vi "Add Initialization Block Diagram Content.vi"(8 "error in (no error)":errorcluster, 10 "Init":T1, 11 "EST Output in":refnum<class "EST Output.lvclass">) -> (0 "error out":errorcluster, 3 "EST Output out":refnum<class "EST Output.lvclass">)   [LabVIEW 2025, in "EST Output.lvclass"]
uses:
  EST Output.lvclass
  VI/VI/Init.Refs.ctl
  <vilib>/Utility/miscctls.llb/LVPointTypeDef.ctl
  <vilib>/_script/New VI Object TypeDefs/NewVIObject_LVRelativePositionTypeDef.ctl
  <vilib>/_script/New VI Object TypeDefs/NewVIObject_LVRelativeDirectionTypeDef.ctl
  <vilib>/Utility/miscctls.llb/LVPoint32TypeDef.ctl
  EST Output.lvclass/EST Output.ctl
  Signal/Read Signal Name.vi
  Read Memory Template Path.vi
  Read Load Path.vi
  VI/Structures/Structures.lvclass
  VI/VI/VI.lvclass
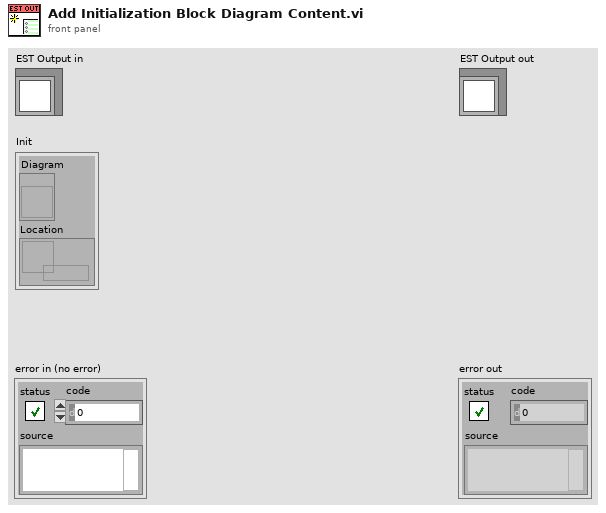
[diagram p1: front panel]
types:
  T1 = typedef "VI.lvclass/Init.Refs.ctl" = cluster{"Diagram":refnum<vi>, "Location":refnum<data-value>}
  T2 = typedef "NewVIObject_LVRelativePositionTypeDef.ctl" = cluster{"Refnum":refnum<vi>, "Relative Direction":T3, "Point32":T4}
  T3 = typedef "NewVIObject_LVRelativeDirectionTypeDef.ctl" = enum32{"Right", "Left", "Top", "Bottom", "Top Right", "Top Left", "Bottom Right", "Bottom Left"}
  T4 = typedef "LVPoint32TypeDef.ctl" = cluster{"Horizontal":i32, "Vertical":i32}
  T5 = typedef "LVPointTypeDef.ctl" = cluster{"Horizontal":i16, "Vertical":i16}
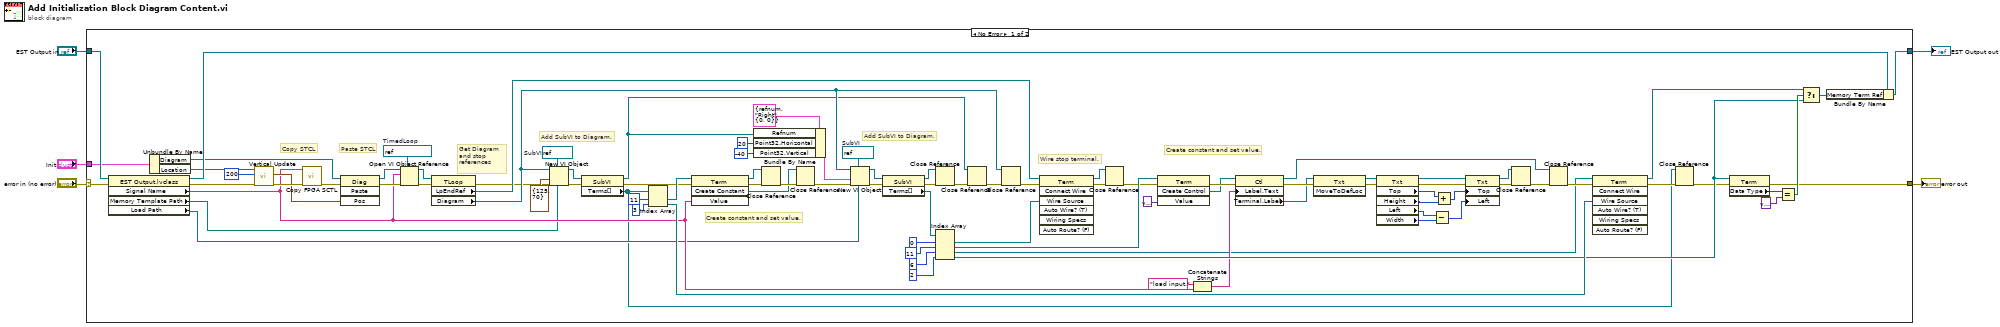
[diagram p0: block diagram]
diagram:
  n1 = case shown="No Error" "error in (no error)" {
    selector: "error in (no error)" -> [w59 w99]
    tunnel: "EST Output in" -> [w64 w100]
    tunnel: [w7 w99] -> w3
    tunnel: [w6 w100] -> w2
    tunnel: "Init" -> [w61 _]
    frame No Error {
      w55 = refnum<vi> refnum  # TimedLoop
      w89 = refnum<vi> refnum  # SubVI
      w84 = refnum<vi> refnum  # SubVI
      # "Create constant and set value."
      # "Wire stop terminal."
      # "Create constant and set value."
      # "Add SubVI to Diagram."
      # "Add SubVI to Diagram."
      # "Get Diagram and stop references"
      # "Paste STCL"
      # "Copy STCL"
      n2 = property class="EST Output.lvclass"(reference=w64, error in=w59) -> (reference out=w63:refnum<class "EST Output.lvclass">, error out=w45:errorcluster, "Signal Name"=w50:string, "Memory Template Path"=w42:path, "Load Path"=w43:path)
      n3 = Unbundle By Name(w61) -> ("Diagram"=w26:refnum<vi>, "Location"=w44:refnum<data-value>)
      n4 = call "Vertical Update.vi"("error in (no error)"=w45, "Vertical Change"=i16 200, "Location"=w44) -> ("error out"=w58:errorcluster, "location out"=w56:T5)  [unwired: 6 in, 1 out]
      n5 = call "Copy FPGA SCTL.vi"("error in (no error)"=w58, "SCTL Name"=w50) -> ("error out"=w57:errorcluster)  [unwired: 9 in]
      n6 = invoke class="Diag" method="Paste"(reference=w26, error in=w57, "Pos"=w56) -> (reference out=w54:refnum<vi>, error out=w53:errorcluster)  [unwired: 1 in, 2 out]
      n7 = Open VI Object Reference(7:w55, 8:w53, 10:w50, 11:w54) -> (0:w52:errorcluster, 3:w51:refnum<vi>)
      n8 = property class="TLoop"(reference=w51, error in=w52) -> (error out=w27:errorcluster, "LpEndRef"=w83:refnum<vi>, "Diagram"=w31:refnum<vi>)  [unwired: 1 out]
      n9 = New VI Object(vi object class=w84, owner refnum=w31, position/next to=T5 {"Horizontal"=125, "Vertical"=70} ("location"), 6:w42, 8:w27) -> (object refnum=w87:refnum<vi>, 0:w88:errorcluster)  [unwired: 3 in]
      n10 = property class="SubVI"(reference=w87, error in=w88) -> (reference out=w30:refnum<vi>, error out=w34:errorcluster, "Terms[]"=w36:refnum<vi>[])
      n11 = Index Array(array=w36, index #1=11 ("index"), index #2=3 ("index")) -> (element #1=w81:refnum<vi>, element #2=w82:refnum<vi>)
      n12 = invoke class="Term" method="Create Constant"(reference=w81, error in=w34, "Value"=w50) -> (reference out=w80:refnum<vi>, error out=w79:errorcluster, "Create Constant"=w76:refnum<vi>)  [unwired: 1 in, 1 out]
      n13 = Bundle By Name(cluster=T2 {"Refnum"=refnum, "Relative Direction"=enum."Right", "Point32"={"Horizontal"=0, "Vertical"=0}} ("Relative Position"), "Refnum"=w30, "Point32.Horizontal"=20, "Point32.Vertical"=-40) -> (w48:T2)
      n14 = Close Reference(reference=w80, error in (no error)=w79) -> (error out=w78:errorcluster)
      n15 = Close Reference(reference=w76, error in (no error)=w78) -> (error out=w77:errorcluster)
      n16 = New VI Object(vi object class=w89, owner refnum=w31, position/next to=w48, 6:w43, 8:w77) -> (object refnum=w91:refnum<vi>, 0:w90:errorcluster)  [unwired: 3 in]
      n17 = property class="SubVI"(reference=w91, error in=w90) -> (reference out=w75:refnum<vi>, error out=w74:errorcluster, "Terms[]"=w94:refnum<vi>[])
      n18 = Close Reference(reference=w75, error in (no error)=w74) -> (error out=w35:errorcluster)
      n19 = Index Array(array=w94, index #1=0 ("index"), index #2=11 ("index"), index #3=6 ("index"), index #4=2 ("index")) -> (element #1=w73:refnum<vi>, element #2=w72:refnum<vi>, element #3=w23:refnum<vi>, element #4=w67:refnum<vi>)
      n20 = Close Reference(reference=w30, error in (no error)=w35) -> (error out=w33:errorcluster)
      n21 = Close Reference(reference=w31, error in (no error)=w33) -> (error out=w32:errorcluster)
      n22 = invoke class="Term" method="Connect Wire"(reference=w83, error in=w32, "Wire Source"=w73) -> (reference out=w41:refnum<vi>, error out=w40:errorcluster)  [unwired: 4 in, 5 out]
      n23 = Close Reference(reference=w41, error in (no error)=w40) -> (error out=w39:errorcluster)
      n24 = invoke class="Term" method="Create Control"(reference=w72, error in=w39, "Value"=variant) -> (error out=w96:errorcluster, "Create Control"=w95:refnum<vi>)  [unwired: 1 in, 2 out]
      n25 = Concatenate Strings("load input." ("string"), w50) -> (w29:string)
      n26 = property class="Ctl"(reference=w95, error in=w96, "Label.Text"=w29) -> (reference out=w12:refnum<vi>, error out=w22:errorcluster, "Terminal.Label"=w21:refnum<vi>)
      n27 = invoke class="Txt" method="MoveToDefLoc"(reference=w21, error in=w22) -> (reference out=w20:refnum<vi>, error out=w19:errorcluster)  [unwired: 1 in, 1 out]
      n28 = property class="Txt"(reference=w20, error in=w19) -> (reference out=w16:refnum<vi>, error out=w15:errorcluster, "Top"=w18:i32, "Height"=w17:u32, "Left"=w10:i32, "Width"=w9:u32)
      n29 = Subtract(x=w10, y=w9) -> (x-y=w8:u32)
      n30 = Add(x=w18, y=w17) -> (x+y=w14:u32)
      n31 = property class="Txt"(reference=w16, error in=w15, "Top"=w14, "Left"=w8) -> (reference out=w11:refnum<vi>, error out=w13:errorcluster)
      n32 = Close Reference(reference=w11, error in (no error)=w13) -> (error out=w25:errorcluster)
      n33 = Close Reference(reference=w12, error in (no error)=w25) -> (error out=w24:errorcluster)
      n34 = invoke class="Term" method="Connect Wire"(reference=w23, error in=w24, "Wire Source"=w82) -> (reference out=w66:refnum<vi>, error out=w38:errorcluster)  [unwired: 4 in, 5 out]
      n35 = Close Reference(reference=w36, error in (no error)=w38) -> (error out=w37:errorcluster)
      n36 = property class="Term"(reference=w67, error in=w37) -> (error out=w7:errorcluster, "Data Type"=w70:variant)  [unwired: 1 out]
      n37 = Equal?(x=w70, y=variant ("x")) -> (x = y?=w68:bool)
      n38 = Select(t=w66, s=w68, f=w67) -> (s? t:f=w62:refnum<vi>)
      n39 = Bundle By Name(cluster=w63, "Memory Term Ref"=w62) -> (w6:refnum<class "EST Output.lvclass">)
    }
    frame Error {
    }
  }
  "error out" <- w3
  "EST Output out" <- w2
